vi "CameraSerialController_2024-04-21.vi"() -> (4 "图像时间戳":u32=16532020 format="%_32g")   [LabVIEW 2015]
uses:
  <vilib>/Instr/_visa.llb/VISA Configure Serial Port (Instr).vi
  MVCAMSDK.dll
  <vilib>/Analysis/NI_AALBase.lvlib
panel:
  out "实时循环时间":u32=16532020 format="%_32g"
  in  "平移前进 2":T1=TRUE
  in  "平移计数 2":u16
  in  "平移一次脉冲数 2":u16=20
  out "连接的字符串 2":string
  out "平移信号曲线 2":cluster{"Locations":dbl[], "Amplitudes":dbl[]}[](graph)
  out "光强图 4":dbl[](graph)
  out "variance 4":dbl caption="方差" format="%0.2f"
  out "光强图 3":dbl[](graph)
  out "variance 3":dbl caption="方差" format="%0.2f"
  out "连接的字符串":string
  out "转动信号曲线":cluster{"Locations":dbl[], "Amplitudes":dbl[]}[](graph)
  in  "平移回退":T1=TRUE
  in  "转动回退":T1=TRUE
  in  "转动计数":u16
  in  "转动一次脉冲数":u16=20
  in  "转动前进":T1=TRUE
  in  "平移一次脉冲数":u16=20
  in  "平移计数":u16
  out "variance 2":dbl caption="方差" format="%0.2f"
  in  "flow control (0:none)":u16(ring) caption="流控制（0:无）" items=["无", "XON/XOFF", "RTS/CTS", "XON/XOFF & RTS/CTS", "DTR/DSR", "XON/XOFF & DTR/DSR"]
  in  "stop bits (10: 1 bit)":u16=10 caption="停止位（10: 1位）"
  in  "奇偶 (0:none)":enum16{"None", "Odd", "Even", "Mark", "Space"}(ring) caption="奇偶（0:无）"
  in  "数据比特(默认8)":u16(ring)=8 items=["5"=5, "6"=6, "7"=7, "8"=8]
  in  "波特率(默认9600)":u32=9600
  in  "端口":refnum<visa-resource-name>="COM1"
  in  "平移前进":T1=TRUE
  out "泰伯距离数值":dbl[](array[numeric])=[15.393849374426454, 15.239052716055017, 15.197063981826837, 15.002070246239633]
  out "Locations":dbl[](array[numeric])=[10.438621227921368, 25.832470602347822, 41.07152331840284, 56.268587300229676, 71.27065754646931] caption="上面图像曲线波峰位置"
  out "平移信号曲线":cluster{"Locations":dbl[], "Amplitudes":dbl[]}[](graph)
  out "光强图 2":dbl[](graph)
  out "variance":dbl caption="方差" format="%0.2f"
  out "相机图像":T2(plugin-control)
  out "光强图":dbl[](graph)
  out "帧速":u32
  out "帧间耗时\n单位：（0.1ms）":u32
  in  "相机枚举":T3(ring)
  in  "自动曝光模式":bool=TRUE caption="软触发"
  in  "手动曝光模式":bool caption="软触发"
  in  "曝光时间，单位微秒":dbl=11000.0 format="%#_6f"
  in  "硬触发模式":bool caption="软触发"
  in  "软触发模式":bool caption="软触发"
  in  "连续模式":bool caption="软触发"
  in  "软触发一帧":bool caption="软触发"
  in  "读取自定义数据":bool
  out "从相机中读出的字符串(32字节)":string
  in  "写入自定义数据":bool
  in  "要写入相机的字符串(32字节)":string
  in  "拍照":bool
  in  "相机参数":bool=TRUE
  in  "Stop":bool
  in  "激活预览":bool=TRUE
  out "Image":T2(plugin-control)
  # "相机原生分辨率设置"
  # "写入自定义数据"
  # "触发设置"
  # "曝光设置"
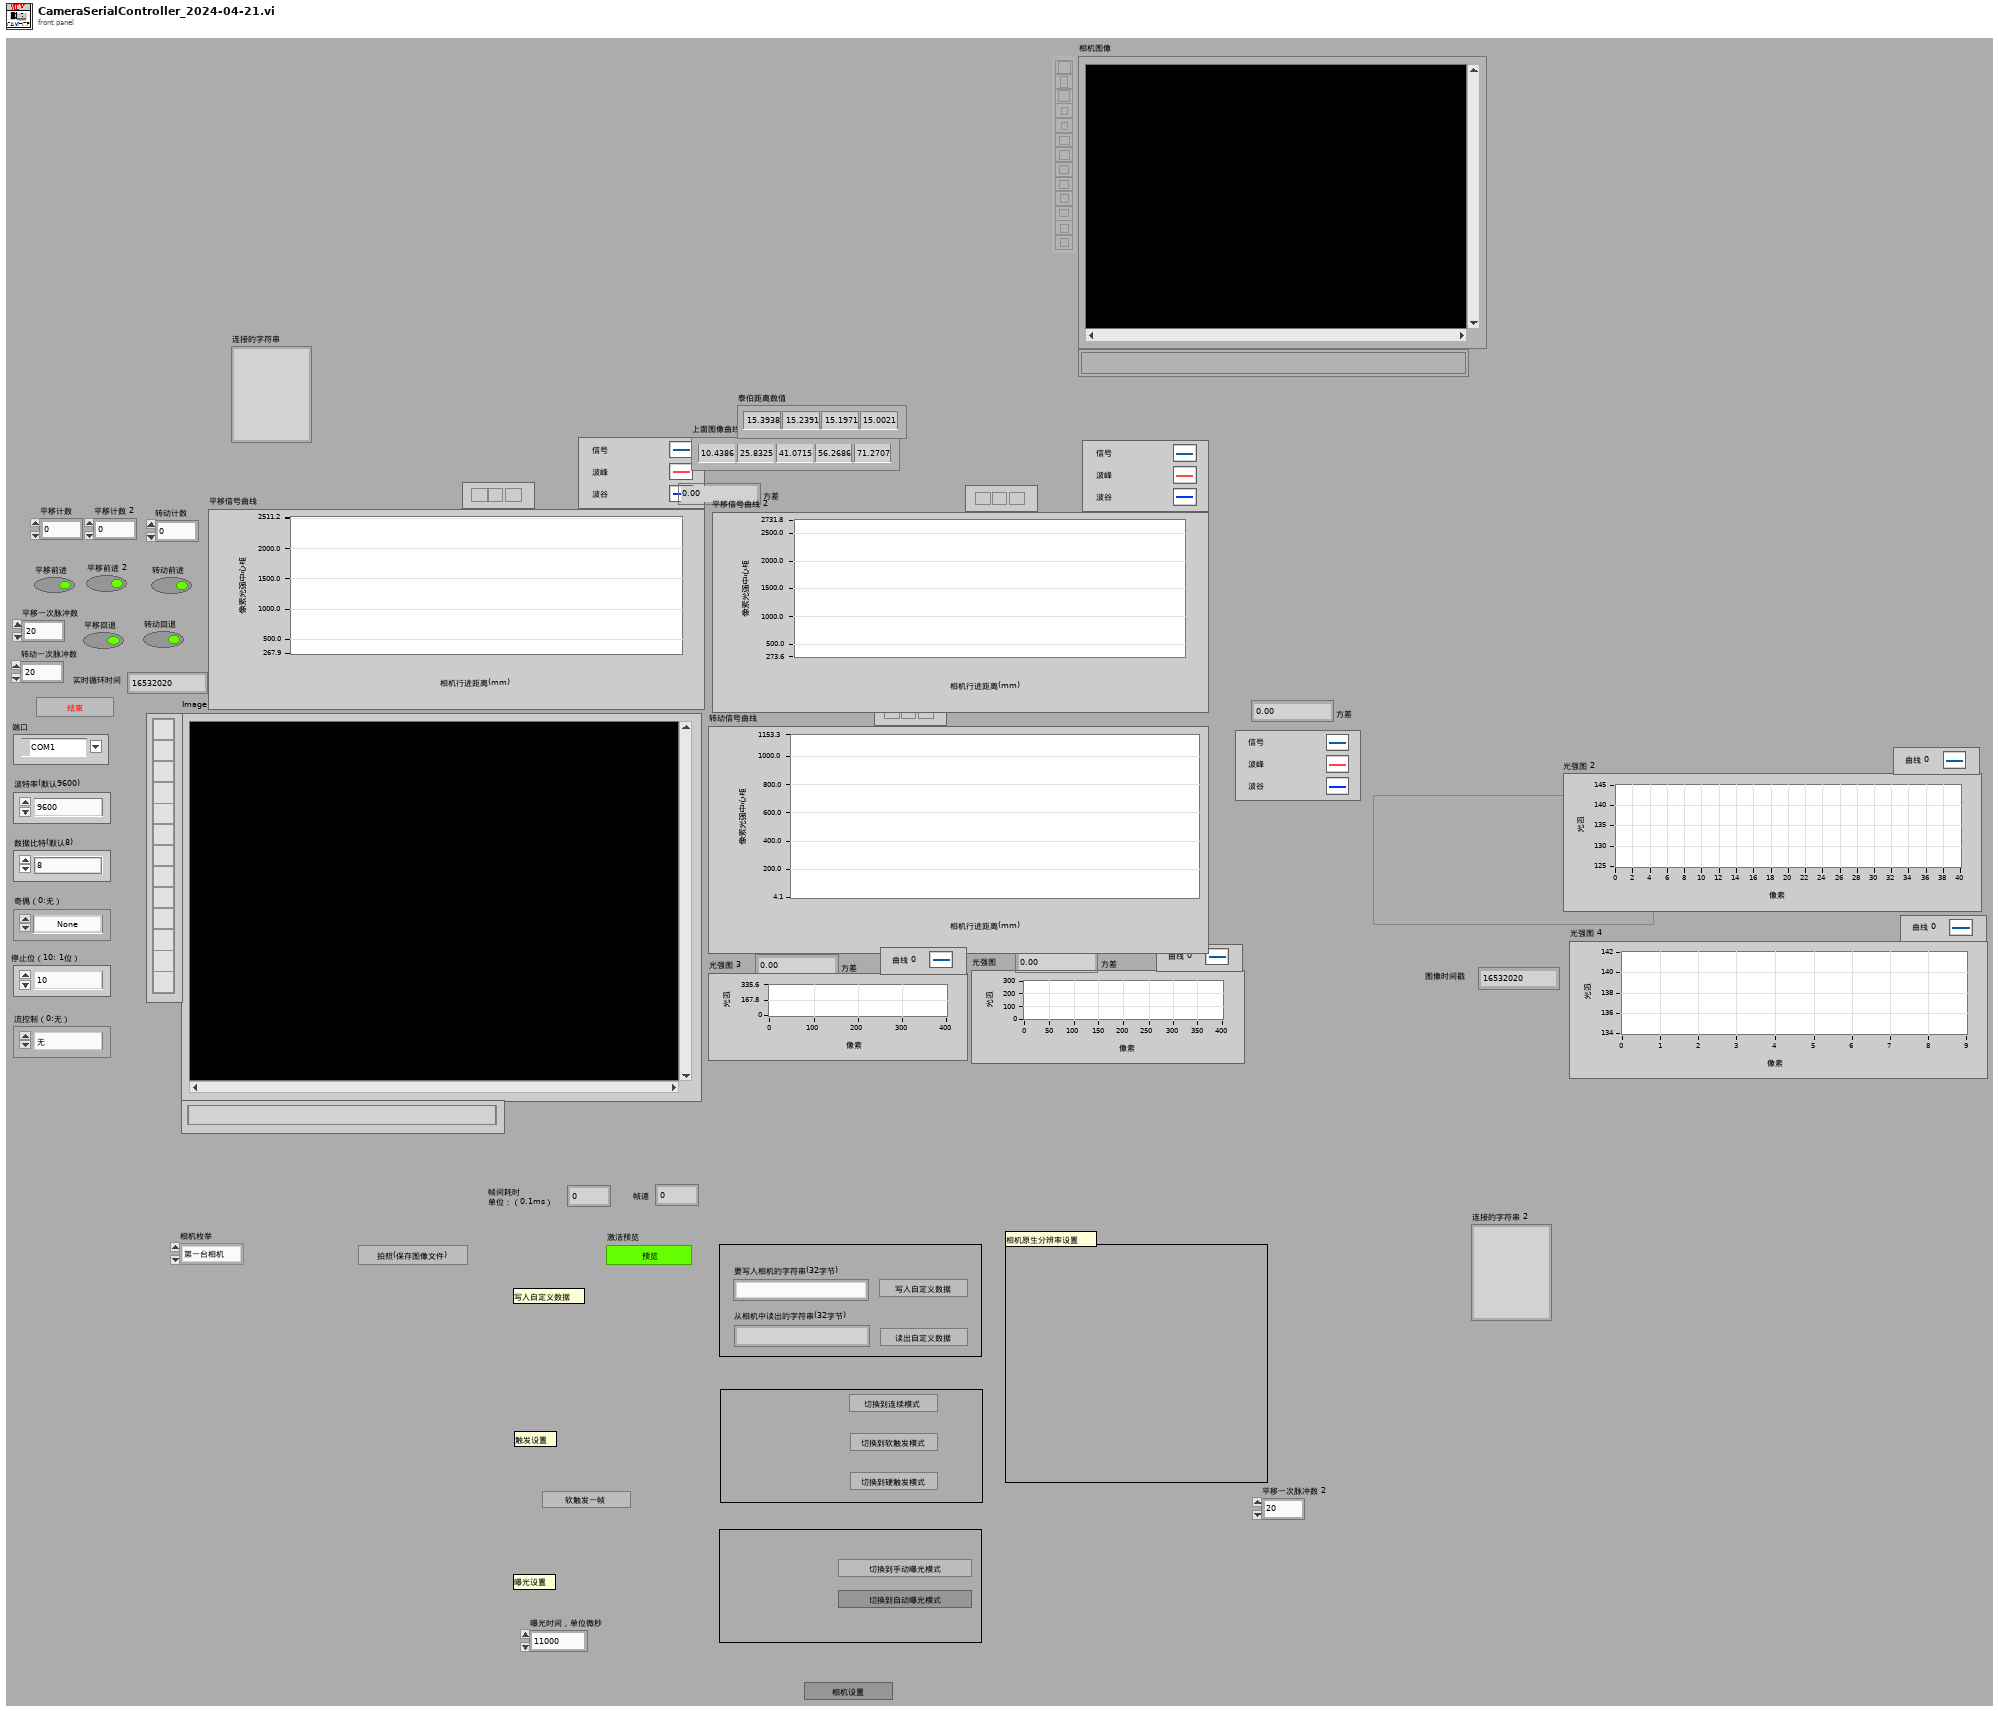
[diagram p1: front panel]
types:
  T1 = typedef "控件 1.ctl" = bool
  T2 = typedef "IMAQ Image.ctl" = refnum<image>
  T3 = enum16{"第一台相机", "第二台相机", "第三台相机", "第四台相机", "第五台相机"}
  T4 = typedef "Image Type" = u32
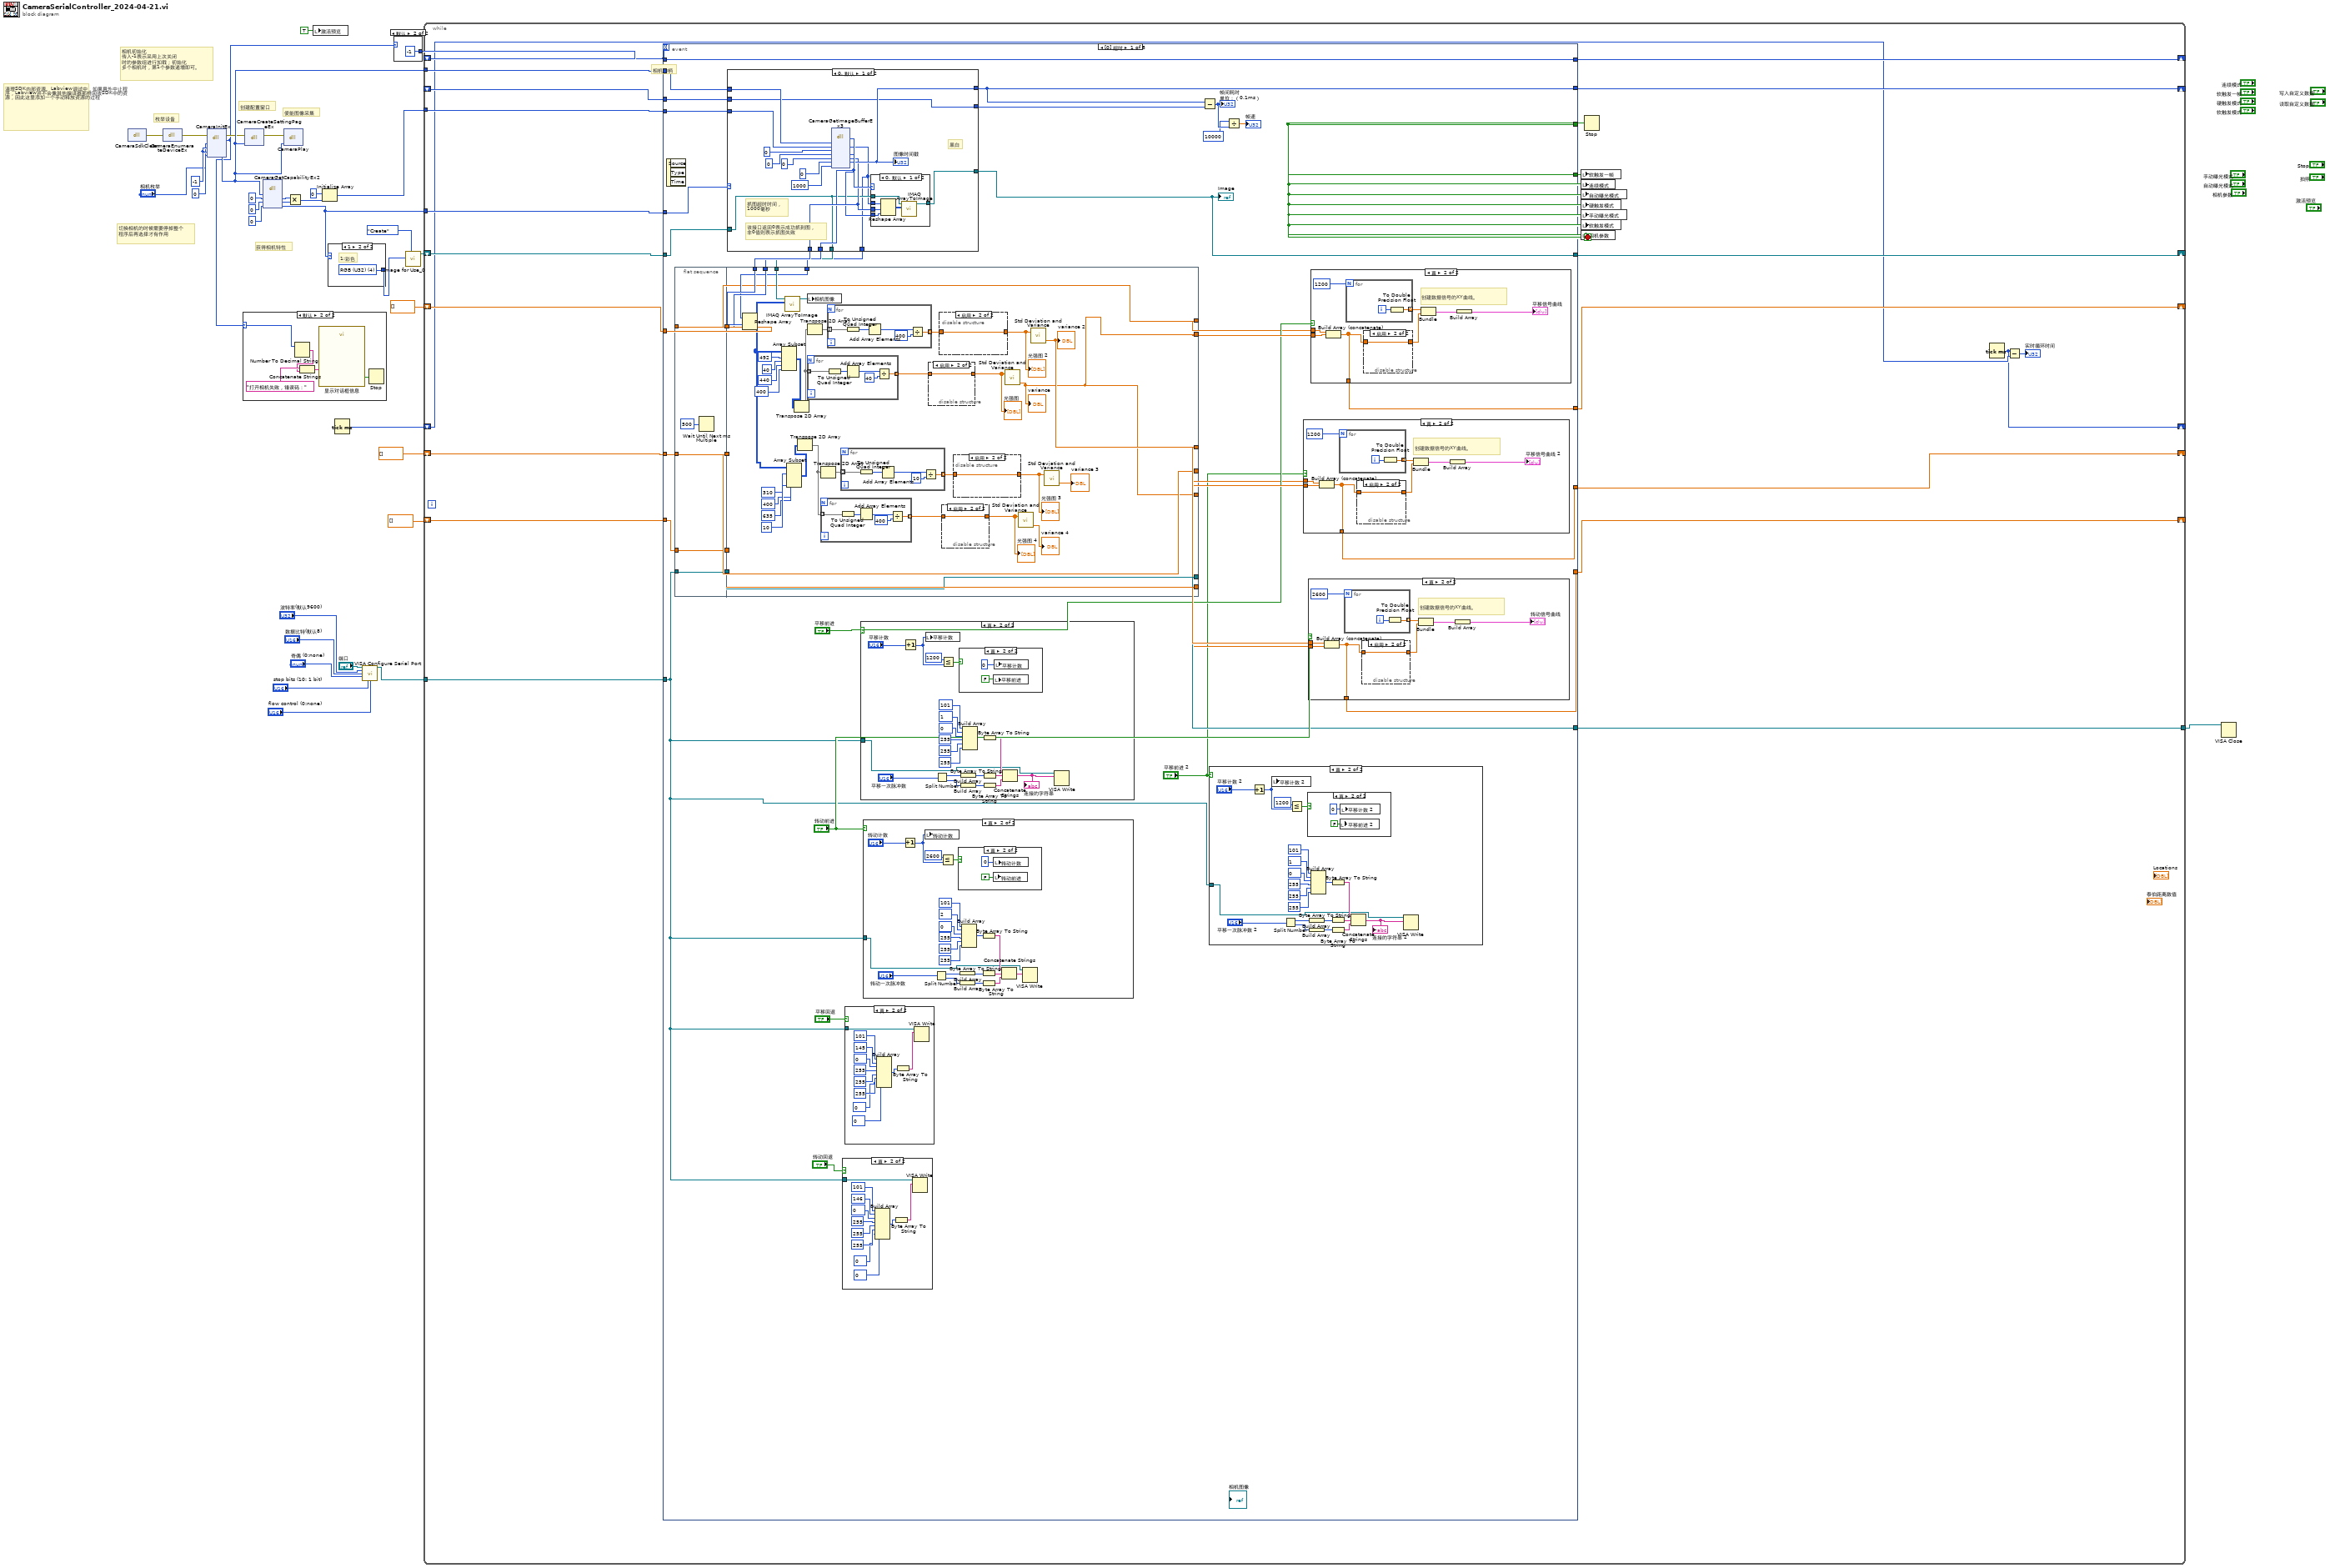
[diagram p0: block diagram]
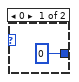
[diagram p2: hidden frame]
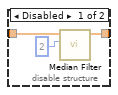
[diagram p7: hidden frame]
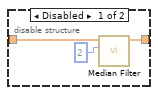
[diagram p8: hidden frame]
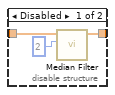
[diagram p9: hidden frame]
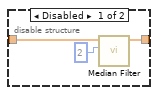
[diagram p10: hidden frame]
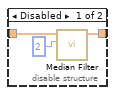
[diagram p11: hidden frame]
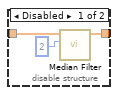
[diagram p13: hidden frame]
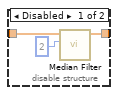
[diagram p15: hidden frame]
diagram:
  w32 = -1
  # "切换相机的时候需要停掉整个\n程序后再选择才有作用"
  # "清理SDK内部资源。Labview调试中，如果意外中止程序，Labview并不会像其他编译器那样回收SDK中的资源，因此这里添加一个手动释放资源的过程"
  # "使能图像采集"
  # "获得相机特性"
  # "创建配置窗口"
  # "相机初始化\n传入-1表示采用上次关闭\n时的参数组进行加载；初始化\n多个相机时，第1个参数递增即可。"
  # "枚举设备"
  n1 = dll-call lib="MVCAMSDK.dll" fn="CameraSdkClean"() -> (error out=w33:errorcluster)  [unwired: 4 in, 1 out]
  n2 = dll-call lib="MVCAMSDK.dll" fn="CameraEnumerateDeviceEx"(error in=w33) -> (error out=w30:errorcluster)  [unwired: 3 in, 1 out]
  n3 = dll-call lib="MVCAMSDK.dll" fn="CameraInitEx"(error in=w30, "相机索引值"="相机枚举", "参数加载方式"=w32, "要加载的参数组索引"=w32, "相机句柄"=0) -> (error out=w19:errorcluster, "返回类型"=w14:i32, "相机句柄"=w21:i32)  [unwired: 5 in, 1 out]
  n4 = case shown="默认" w14 {
    selector: w14 -> [_ w39]
    frame 0 {
    }
    frame Default {
      n5 = Number To Decimal String(number=w39) -> (decimal integer string=w36:string)  [unwired: 1 in]
      n6 = Concatenate Strings("打开相机失败，错误码：" ("字符串"), w36) -> (w38:string)
      n7 = call "显示对话框信息"("Message"=w38) -> ("结束"=w40:bool)  [unwired: 9 in, 1 out]
      n8 = Stop(stop? (T)=w40) -> ()
    }
  }
  n9 = dll-call lib="MVCAMSDK.dll" fn="CameraCreateSettingPageEx"(error in=w19, "相机句柄"=w21) -> (error out=w22:errorcluster)  [unwired: 4 in, 1 out]
  n10 = dll-call lib="MVCAMSDK.dll" fn="CameraGetCapabilityEx2"("相机句柄"=w21, "图像最大宽度"=0, "图像最大高度"=0, "是否是彩色相机(返回0:黑白;1:彩色)"=0) -> ("图像最大宽度"=w24:i32, "图像最大高度"=w23:i32, "是否是彩色相机(返回0:黑白;1:彩色)"=w18:i32)  [unwired: 5 in, 2 out]
  n11 = dll-call lib="MVCAMSDK.dll" fn="CameraPlay"(error in=w22, "相机句柄"=w21) -> ()  [unwired: 4 in, 2 out]
  n12 = Multiply(x=w24, y=w23) -> (x*y=w28:i32)
  n13 = local write "激活预览"(TRUE ("激活预览")) -> ()
  n14 = Initialize Array(0, w28) -> (w20:i32[])
  n15 = case shown="1" w18 {
    tunnel: [_ w41] -> w34
    frame 0, Default {
      # "0:黑白;"
    }
    frame 1 {
      w41 = T4 4 items=["Grayscale (U8)", "Grayscale (I16)", "Grayscale (SGL)", "Complex (CSG)", "RGB (U32)", "HSL (U32)", "RGB (U64)", "Grayscale (U16)"] ("Image Type")
      # "1:彩色"
    }
  }
  n16 = Tick Count (ms)() -> (millisecond timer value=w1:u32)
  n17 = call-poly "VISA Configure Serial Port"("VISA resource name"="端口", "baud rate (9600)"="波特率(默认9600)", "data bits (8)"="数据比特(默认8)", "parity (0:none)"="奇偶 (0:none)", "stop bits (10: 1 bit)"="stop bits (10: 1 bit)", "flow control (0:none)"="flow control (0:none)") -> ("VISA resource name out"=w6:refnum<visa-resource-name>)  [unwired: 8 in, 1 out]
  n18 = case shown="默认" w14 {
    tunnel: [0 -1] -> w13
    frame 0 {
    }
    frame Default {
    }
  }
  n19 = call "Image for Use_0.vi"("Command"=enum16{"Create", "Use", "Copy in", "Dispose"}."Create", "Image Type"=w34) -> ("Image out"=w17:T2)  [unwired: 8 in, 1 out]
  n20 = while {
    tunnel: w21 -> [w62]
    tunnel: w20 -> [w64]
    tunnel: w18 -> [w65]
    shift-right: [w61] -> _
    shift-left: w13 -> [w60]
    shift-right: [w58] -> _
    shift-left: w17 -> [w63]
    shift-right: [w57] -> _
    shift-left: _ -> [w56]
    tunnel: w6 -> [w54]
    tunnel: [w53] -> w5
    shift-right: [w51] -> _
    shift-left: dbl[] [] -> [w52]
    shift-right: [w50] -> _
    shift-left: dbl[] [] -> [w49]
    shift-right: [w47] -> _
    shift-left: dbl[] [] -> [w48]
    shift-right: [w44] -> _
    shift-left: w1 -> [w45]
    stop <- w55 stop-if-true
    # "相机句柄"
    n21 = event shown="[0] 超时" {
      selector: _ -> [_ _ _ _ _ _ _ _]
      dyn-events: _ -> [_ _ _ _ _ _ _ _]
      timeout: w60 -> [_ _ _ _ _ _ _ _]
      tunnel: [_ _ _ _ _ _ _ TRUE] -> w55
      tunnel: w64 -> [w103 _ _ _ _ _ _ _]
      tunnel: w65 -> [w102 _ _ _ _ _ _ _]
      tunnel: w62 -> [w104 _ w371 w389 w404 _ w418 w438]
      tunnel: w63 -> [w101 w364 w370 w388 w403 w408 w417 w436]
      tunnel: [w100 w365 w372 w390 w405 w409 w419 w439] -> w61
      tunnel: w60 -> [w100 _ w372 w390 w405 w409 w419 w439]
      tunnel: [_ _ _ _ _ _ _ FALSE] -> w59
      tunnel: [w99 w364 w370 w388 w403 w408 w417 w436] -> w58
      tunnel: [w96 w363 w369 w387 w402 w407 w416 w435] -> w57
      tunnel: w56 -> [w98 w363 w369 w387 w402 w407 w416 w435]
      tunnel: w54 -> [w66 _ _ _ _ _ _ _]
      tunnel: [w77 _ _ _ _ _ _ _] -> w53
      tunnel: w52 -> [w83 _ _ _ _ _ _ _]
      tunnel: [w86 _ _ _ _ _ _ _] -> w51
      tunnel: [w85 _ _ _ _ _ _ _] -> w50
      tunnel: w49 -> [w79 _ _ _ _ _ _ _]
      tunnel: [w74 _ _ _ _ _ _ _] -> w47
      tunnel: w48 -> [w71 _ _ _ _ _ _ _]
      event Timeout {
        n22 = event-data() -> ()  [unwired: 1 in, 3 out]
        n23 = flat-sequence {
          tunnel: w83 -> [w147]
          tunnel: [w147] -> w82
          tunnel: [w145] -> w80
          tunnel: w79 -> [w145]
          tunnel: [w144] -> w78
          tunnel: w66 -> [w144]
          tunnel: w71 -> [w143]
          tunnel: [w143] -> w70
          tunnel: w92 -> [w182]
          tunnel: w91 -> [w181]
          tunnel: w90 -> [w180]
          tunnel: w89 -> [w179]
          tunnel: [w149] -> w75
          tunnel: [w169] -> w68
          tunnel: w82 -> [w169]
          tunnel: [w168] -> w81
          tunnel: w80 -> [w168]
          tunnel: [w167] -> w77
          tunnel: w78 -> [w167]
          tunnel: [w151] -> w76
          tunnel: [w149] -> w73
          tunnel: w70 -> [w150]
          tunnel: [w150] -> w69
          frame #0 {
            n24 = Wait Until Next ms Multiple(millisecond multiple=u32 500 ("毫秒倍数")) -> ()  [unwired: 1 out]
          }
          frame #1 {
            n25 = Reshape Array(w179, w182, w181) -> (w156:u8[][])
            n26 = Array Subset(array=w156, index (row)=492 ("索引"), length (row)=40 ("长度"), index (col)=440 ("长度"), length (col)=400 ("索引")) -> (w153:u8[][])
            n27 = call "IMAQ ArrayToImage"("Image Pixels (U8)"=w156, "Image"=w180) -> ("Image Out"=w183:T2)  [unwired: 8 in, 1 out]
            n28 = Array Subset(array=w156, index (row)=310 ("索引"), length (row)=400 ("长度"), index (col)=635 ("长度"), length (col)=10 ("索引")) -> (w155:u8[][])
            n29 = Transpose 2D Array(2D array=w153) -> (transposed array=w152:u8[][])
            n30 = Transpose 2D Array(2D array=w155) -> (transposed array=w154:u8[][])
            n31 = local write "相机图像"(w183) -> ()
            n32 = Transpose 2D Array(2D array=w152) -> (transposed array=w176:u8[][])
            n33 = for {
              tunnel: w152 -> [w214] mode=indexing
              tunnel: [w212] -> w178 mode=indexing
              n34 = To Unsigned Quad Integer(1:w214) -> (0:w213:u64[])
              n35 = Add Array Elements(numeric array=w213) -> (sum=w215:u64)
              n36 = Divide(x=w215, y=u64 40) -> (x/y=w212:dbl)
            }
            n37 = Transpose 2D Array(2D array=w154) -> (transposed array=w160:u8[][])
            n38 = for {
              tunnel: w154 -> [w196] mode=indexing
              tunnel: [w194] -> w158 mode=indexing
              n39 = To Unsigned Quad Integer(1:w196) -> (0:w195:u64[])
              n40 = Add Array Elements(numeric array=w195) -> (sum=w197:u64)
              n41 = Divide(x=w197, y=u64 400) -> (x/y=w194:dbl)
            }
            n42 = for {
              tunnel: w176 -> [w205] mode=indexing
              tunnel: [w203] -> w177 mode=indexing
              n43 = To Unsigned Quad Integer(1:w205) -> (0:w204:u64[])
              n44 = Add Array Elements(numeric array=w204) -> (sum=w206:u64)
              n45 = Divide(x=w206, y=u64 400) -> (x/y=w203:dbl)
            }
            n46 = for {
              tunnel: w160 -> [w187] mode=indexing
              tunnel: [w185] -> w159 mode=indexing
              n47 = To Unsigned Quad Integer(1:w187) -> (0:w186:u64[])
              n48 = Add Array Elements(numeric array=w186) -> (sum=w188:u64)
              n49 = Divide(x=w188, y=u64 10) -> (x/y=w185:dbl)
            }
            n50 = disable-structure shown="启用" {
              disable-tunnel: w178 -> [w218 w219]
              disable-tunnel: [w216 w219] -> w175
              frame Disabled {
                n51 = call <vilib>:"Median Filter.vi"("left rank"=2, "X"=w218) -> ("Filtered X"=w216:dbl[])  [unwired: 8 in, 1 out]
              }
              frame Enabled {
              }
            }
            "光强图" <- w175
            n52 = disable-structure shown="启用" {
              disable-tunnel: w177 -> [w209 w210]
              disable-tunnel: [w207 w210] -> w174
              frame Disabled {
                n53 = call <vilib>:"Median Filter.vi"("left rank"=2, "X"=w209) -> ("Filtered X"=w207:dbl[])  [unwired: 8 in, 1 out]
              }
              frame Enabled {
              }
            }
            "光强图 2" <- w174
            n54 = disable-structure shown="启用" {
              disable-tunnel: w158 -> [w200 w201]
              disable-tunnel: [w198 w201] -> w161
              frame Disabled {
                n55 = call <vilib>:"Median Filter.vi"("left rank"=2, "X"=w200) -> ("Filtered X"=w198:dbl[])  [unwired: 8 in, 1 out]
              }
              frame Enabled {
              }
            }
            "光强图 4" <- w161
            n56 = disable-structure shown="启用" {
              disable-tunnel: w159 -> [w191 w192]
              disable-tunnel: [w189 w192] -> w162
              frame Disabled {
                n57 = call <vilib>:"Median Filter.vi"("left rank"=2, "X"=w191) -> ("Filtered X"=w189:dbl[])  [unwired: 8 in, 1 out]
              }
              frame Enabled {
              }
            }
            "光强图 3" <- w162
            n58 = call <vilib>:"Std Deviation and Variance.vi"("X"=w175) -> ("variance"=w149:dbl)  [unwired: 1 in, 2 out]
            "variance" <- w149
            n59 = call <vilib>:"Std Deviation and Variance.vi"("X"=w161) -> ("variance"=→"variance 4":dbl)  [unwired: 1 in, 2 out]
            n60 = call <vilib>:"Std Deviation and Variance.vi"("X"=w174) -> ("variance"=w151:dbl)  [unwired: 1 in, 2 out]
            "variance 2" <- w151
            n61 = call <vilib>:"Std Deviation and Variance.vi"("X"=w162) -> ("variance"=→"variance 3":dbl)  [unwired: 1 in, 2 out]
          }
        }
        n62 = case shown="0, 默认" w102 {
          tunnel: w103 -> [w332 w355]
          tunnel: w101 -> [w319 w354]
          tunnel: w104 -> [w324 w353]
          tunnel: [w325 w343] -> w99
          tunnel: [w323 w342] -> w96
          tunnel: w98 -> [w322 w341]
          tunnel: [w322 w341] -> w97
          tunnel: [w321 _] -> w92
          tunnel: [w320 _] -> w91
          tunnel: [w319 _] -> w90
          tunnel: [w318 _] -> w89
          frame 0, Default {
            # "黑白"
            # "该接口返回0表示成功抓到图，\n非0值则表示抓图失败"
            # "抓图超时时间，\n1000毫秒"
            n63 = dll-call lib="MVCAMSDK.dll" fn="CameraGetImageBufferEx3"("相机句柄"=w324, "图像数据缓冲区"=w332, "图像输出格式(0:8位灰度;1:24位彩色;2:32位彩色，3：BGR24彩色 4：BGRA32位彩色)"=0, "图像宽度"=0, "图像高度"=0, "时间戳(单位为100微秒)"=0, "抓图超时时间(毫秒)"=1000) -> ("返回类型"=w327:i32, "图像数据缓冲区"=w318:u8[], "图像宽度"=w320:i32, "图像高度"=w321:i32, "时间戳(单位为100微秒)"=w323:u32)  [unwired: 6 in, 2 out]
            "图像时间戳" <- w323
            n64 = case shown="0, 默认" w327 {
              tunnel: w318 -> [w338 _]
              tunnel: w319 -> [w335 w339]
              tunnel: w321 -> [w337 _]
              tunnel: w320 -> [w336 _]
              tunnel: [w333 w339] -> w325
              frame 0, Default {
                n65 = Reshape Array(w338, w337, w336) -> (w334:u8[][])
                n66 = call "IMAQ ArrayToImage"("Image Pixels (U8)"=w334, "Image"=w335) -> ("Image Out"=w333:T2)  [unwired: 8 in, 1 out]
              }
              frame -12 {
              }
            }
          }
          frame 1 {
            w345 = 0
            w346 = 0
            # "彩色"
            n67 = dll-call lib="MVCAMSDK.dll" fn="CameraGetImageBufferPriorityEx3"("相机句柄"=w353, "图像数据缓冲区"=w355, "图像输出格式(0:8位灰度;1:24位彩色;2:32位彩色)"=4, "图像宽度"=w345, "图像高度"=w346, "时间戳（单位为100微秒）"=0, "抓图超时时间(毫秒)"=1000, "取图优先级(0: 取最旧   1:取最新)"=1) -> ("返回类型"=w347:i32, "图像数据缓冲区"=w350:u32[], "图像宽度"=w348:i32, "图像高度"=w349:i32, "时间戳（单位为100微秒）"=w342:u32)  [unwired: 7 in, 2 out]
            n68 = case shown="0, 默认" w347 {
              tunnel: w350 -> [w360 _]
              tunnel: w354 -> [w359 w362]
              tunnel: w349 -> [w358 _]
              tunnel: w348 -> [w357 _]
              tunnel: w346 -> [_ _]
              tunnel: w345 -> [_ _]
              tunnel: [w356 w362] -> w343
              frame 0, Default {
                n69 = Reshape Array(w360, w358, w357) -> (w361:u32[][])
                n70 = call "IMAQ ArrayToColorImage"("Image Pixels (U32)"=w361, "Image"=w359) -> ("Image Out"=w356:T2)  [unwired: 3 in, 1 out]
              }
              frame -12 {
              }
            }
            n71 = local write "图像时间戳"(w342) -> ()
          }
        }
        "Image" <- w99
        n72 = case shown="真" "转动回退" {
          tunnel: w66 -> [_ w253]
          frame False {
          }
          frame True {
            n73 = Build Array(101, 146, 0, 255, 255, 255, 0, 0) -> (w254:i32[])
            n74 = Byte Array To String(unsigned byte array=w254) -> (string=w252:string)
            n75 = VISA Write(VISA resource name=w253, write buffer=w252) -> ()  [unwired: 1 in, 3 out]
          }
        }
        n76 = case shown="真" "平移回退" {
          tunnel: w66 -> [_ w264]
          frame False {
          }
          frame True {
            n77 = Build Array(101, 145, 0, 255, 255, 255, 0, 0) -> (w265:i32[])
            n78 = Byte Array To String(unsigned byte array=w265) -> (string=w263:string)
            n79 = VISA Write(VISA resource name=w264, write buffer=w263) -> ()  [unwired: 1 in, 3 out]
          }
        }
        n80 = case shown="真" "平移前进" {
          tunnel: w66 -> [_ w298]
          frame False {
          }
          frame True {
            n81 = Increment(x="平移计数") -> (x+1=w296:u16)
            n82 = local write "平移计数"(w296) -> ()
            n83 = Split Number(x="平移一次脉冲数") -> (hi(x)=w306:u8, lo(x)=w305:u8)
            n84 = Less Or Equal?(x=1200, y=w296) -> (x <= y?=w308:bool)
            n85 = case shown="真" w308 {
              frame False {
              }
              frame True {
                n86 = local write "平移前进"(T1 FALSE ("平移前进")) -> ()
                n87 = local write "平移计数"(u16 0 ("平移计数 2")) -> ()
              }
            }
            n88 = Build Array(w306) -> (w304:u8[])
            n89 = Build Array(w305) -> (w303:u8[])
            n90 = Build Array(101, 1, 0, 255, 255, 255) -> (w302:i32[])
            n91 = Byte Array To String(unsigned byte array=w302) -> (string=w301:string)
            n92 = Byte Array To String(unsigned byte array=w304) -> (string=w300:string)
            n93 = Byte Array To String(unsigned byte array=w303) -> (string=w299:string)
            n94 = Concatenate Strings(w301, w300, w299) -> (w295:string)
            "连接的字符串" <- w295
            n95 = VISA Write(VISA resource name=w298, write buffer=w295) -> ()  [unwired: 1 in, 3 out]
          }
        }
        n96 = case shown="真" "转动前进" {
          tunnel: w66 -> [_ w276]
          frame False {
          }
          frame True {
            n97 = Increment(x="转动计数") -> (x+1=w274:u16)
            n98 = local write "转动计数"(w274) -> ()
            n99 = Split Number(x="转动一次脉冲数") -> (hi(x)=w284:u8, lo(x)=w283:u8)
            n100 = Less Or Equal?(x=2600, y=w274) -> (x <= y?=w286:bool)
            n101 = case shown="真" w286 {
              frame False {
              }
              frame True {
                n102 = local write "转动前进"(T1 FALSE ("平移前进")) -> ()
                n103 = local write "转动计数"(u16 0 ("平移计数")) -> ()
              }
            }
            n104 = Build Array(w284) -> (w282:u8[])
            n105 = Build Array(w283) -> (w281:u8[])
            n106 = Build Array(101, 2, 0, 255, 255, 255) -> (w280:i32[])
            n107 = Byte Array To String(unsigned byte array=w280) -> (string=w279:string)
            n108 = Byte Array To String(unsigned byte array=w282) -> (string=w278:string)
            n109 = Byte Array To String(unsigned byte array=w281) -> (string=w277:string)
            n110 = Concatenate Strings(w279, w278, w277) -> (w273:string)
            n111 = VISA Write(VISA resource name=w276, write buffer=w273) -> ()  [unwired: 1 in, 3 out]
          }
        }
        n112 = Subtract(x=w96, y=w97) -> (x-y=w95:u32)
        "帧间耗时\n单位：（0.1ms）" <- w95
        n113 = case shown="真" "平移前进 2" {
          tunnel: w66 -> [_ w108]
          frame False {
          }
          frame True {
            n114 = Increment(x="平移计数 2") -> (x+1=w106:u16)
            n115 = local write "平移计数 2"(w106) -> ()
            n116 = Split Number(x="平移一次脉冲数 2") -> (hi(x)=w116:u8, lo(x)=w115:u8)
            n117 = Less Or Equal?(x=1200, y=w106) -> (x <= y?=w118:bool)
            n118 = case shown="真" w118 {
              frame False {
              }
              frame True {
                n119 = local write "平移前进 2"(T1 FALSE ("平移前进")) -> ()
                n120 = local write "平移计数 2"(u16 0 ("平移计数 2")) -> ()
              }
            }
            n121 = Build Array(w116) -> (w114:u8[])
            n122 = Build Array(w115) -> (w113:u8[])
            n123 = Build Array(101, 1, 0, 255, 255, 255) -> (w112:i32[])
            n124 = Byte Array To String(unsigned byte array=w112) -> (string=w111:string)
            n125 = Byte Array To String(unsigned byte array=w114) -> (string=w110:string)
            n126 = Byte Array To String(unsigned byte array=w113) -> (string=w109:string)
            n127 = Concatenate Strings(w111, w110, w109) -> (w105:string)
            "连接的字符串 2" <- w105
            n128 = VISA Write(VISA resource name=w108, write buffer=w105) -> ()  [unwired: 1 in, 3 out]
          }
        }
        n129 = Divide(x=u32 10000 ("帧间耗时"), y=w95) -> (x/y=→"帧速":dbl)
        n130 = case shown="真" "平移前进 2" {
          tunnel: w69 -> [w128 w131]
          tunnel: w73 -> [_ w129]
          tunnel: [w128 w130] -> w74
          frame False {
          }
          frame True {
            # "创建数据信号的XY曲线。"
            n131 = Build Array (concatenate)(w131, w129) -> (w130:dbl[])
            n132 = for {
              N: i64 1200 ("数值") -> [_]
              tunnel: [w137] -> w135 mode=indexing
              i -> [w138]
              n133 = To Double Precision Float(number=w138) -> (double precision float=w137:dbl)
            }
            n134 = disable-structure shown="启用" {
              disable-tunnel: w130 -> [w140 w142]
              disable-tunnel: [w139 w142] -> w134
              frame Disabled {
                n135 = call <vilib>:"Median Filter.vi"("left rank"=2, "X"=w140) -> ("Filtered X"=w139:dbl[])  [unwired: 8 in, 1 out]
              }
              frame Enabled {
              }
            }
            n136 = Bundle(w135, w134) -> (w132:cluster{dbl[], dbl[]})  [unwired: 1 in]
            n137 = Build Array(w132) -> (→"平移信号曲线 2":cluster{dbl[], dbl[]}[])
          }
        }
        n138 = case shown="真" "转动前进" {
          tunnel: w76 -> [_ w223]
          tunnel: w81 -> [w220 w222]
          tunnel: [w220 w221] -> w85
          frame False {
          }
          frame True {
            # "创建数据信号的XY曲线。"
            n139 = Build Array (concatenate)(w222, w223) -> (w221:dbl[])
            n140 = for {
              N: i64 2600 ("数值") -> [_]
              tunnel: [w229] -> w225 mode=indexing
              i -> [w230]
              n141 = To Double Precision Float(number=w230) -> (double precision float=w229:dbl)
            }
            n142 = disable-structure shown="启用" {
              disable-tunnel: w221 -> [w232 w234]
              disable-tunnel: [w231 w234] -> w226
              frame Disabled {
                n143 = call <vilib>:"Median Filter.vi"("left rank"=2, "X"=w232) -> ("Filtered X"=w231:dbl[])  [unwired: 8 in, 1 out]
              }
              frame Enabled {
              }
            }
            n144 = Bundle(w225, w226) -> (w228:cluster{dbl[], dbl[]})  [unwired: 1 in]
            n145 = Build Array(w228) -> (→"转动信号曲线":cluster{dbl[], dbl[]}[])
          }
        }
        n146 = case shown="真" "平移前进" {
          tunnel: w68 -> [w235 w237]
          tunnel: w75 -> [_ w238]
          tunnel: [w235 w236] -> w86
          frame False {
          }
          frame True {
            # "创建数据信号的XY曲线。"
            n147 = Build Array (concatenate)(w237, w238) -> (w236:dbl[])
            n148 = for {
              N: i64 1200 ("数值") -> [_]
              tunnel: [w244] -> w242 mode=indexing
              i -> [w245]
              n149 = To Double Precision Float(number=w245) -> (double precision float=w244:dbl)
            }
            n150 = disable-structure shown="启用" {
              disable-tunnel: w236 -> [w247 w249]
              disable-tunnel: [w246 w249] -> w241
              frame Disabled {
                n151 = call <vilib>:"Median Filter.vi"("left rank"=2, "X"=w247) -> ("Filtered X"=w246:dbl[])  [unwired: 8 in, 1 out]
              }
              frame Enabled {
              }
            }
            n152 = Bundle(w242, w241) -> (w239:cluster{dbl[], dbl[]})  [unwired: 1 in]
            n153 = Build Array(w239) -> (→"平移信号曲线":cluster{dbl[], dbl[]}[])
          }
        }
      }
      event "激活预览": Value Change {
        n154 = event-data() -> ("NewVal"=w366:bool)  [unwired: 1 in, 5 out]
        n155 = case shown="真" w366 {
          tunnel: [-1 0] -> w365
          frame False {
          }
          frame True {
          }
        }
      }
      event "连续模式", "软触发一帧", "硬触发模式", "软触发模式": Value Change {
        n156 = event-data() -> ("CtlRef"=w374:refnum<vi>)  [unwired: 1 in, 5 out]
        n157 = control-ref of="连续模式"() -> (w376:refnum<vi>)
        n158 = control-ref of="硬触发模式"() -> (w377:refnum<vi>)
        n159 = control-ref of="软触发模式"() -> (w378:refnum<vi>)
        n160 = control-ref of="软触发一帧"() -> (w379:refnum<vi>)
        n161 = Build Array ("创建数组")(w376, w377, w378, w379) -> (w375:refnum<vi>[])
        n162 = Search 1D Array(1D array=w375, element=w374) -> (index of element=w373:i32)  [unwired: 1 in]
        n163 = case shown="1" w373 {
          tunnel: w371 -> [w380 w382 w384 w386]
          frame 0, Default {
            # "连续模式"
            n164 = dll-call lib="MVCAMSDK.dll" fn="CameraSetTriggerMode"("相机句柄"=w380, "模式"=0) -> ()  [unwired: 6 in, 2 out]
          }
          frame 1 {
            # "硬触发模式"
            n165 = dll-call lib="MVCAMSDK.dll" fn="CameraSetTriggerMode"("相机句柄"=w382, "模式"=2) -> ()  [unwired: 6 in, 2 out]
          }
          frame 2 {
            # "软触发模式"
            n166 = dll-call lib="MVCAMSDK.dll" fn="CameraSetTriggerMode"("相机句柄"=w384, "模式"=1) -> ()  [unwired: 6 in, 2 out]
          }
          frame 3 {
            # "软触发一帧"
            n167 = dll-call lib="MVCAMSDK.dll" fn="CameraSoftTrigger"("相机句柄"=w386) -> ()  [unwired: 5 in, 2 out]
          }
        }
      }
      event "手动曝光模式", "自动曝光模式": Value Change {
        n168 = event-data() -> ("CtlRef"=w393:refnum<vi>)  [unwired: 1 in, 5 out]
        n169 = control-ref of="自动曝光模式"() -> (w391:refnum<vi>)
        n170 = control-ref of="手动曝光模式"() -> (w394:refnum<vi>)
        n171 = Build Array ("创建数组")(w394, w391) -> (w395:refnum<vi>[])
        n172 = Search 1D Array(1D array=w395, element=w393) -> (index of element=w392:i32)  [unwired: 1 in]
        n173 = case shown="0, 默认" w392 {
          tunnel: w389 -> [w396 w400]
          frame 0, Default {
            # "手动曝光模式"
            n174 = dll-call lib="MVCAMSDK.dll" fn="CameraSetAeState"("相机句柄"=w396, "曝光模式(0手动，1自动)"=0) -> (error out=w399:errorcluster)  [unwired: 6 in, 1 out]
            n175 = dll-call lib="MVCAMSDK.dll" fn="CameraSetExposureTime"(error in=w399, "相机句柄"=w396, "曝光时间，单位微秒"="曝光时间，单位微秒") -> ()  [unwired: 5 in, 2 out]
          }
          frame 1 {
            # "自动曝光模式"
            n176 = dll-call lib="MVCAMSDK.dll" fn="CameraSetAeState"("相机句柄"=w400, "曝光模式(0手动，1自动)"=1) -> ()  [unwired: 6 in, 2 out]
          }
        }
      }
      event "相机参数": Value Change {
        n177 = event-data() -> ()  [unwired: 1 in, 6 out]
        n178 = dll-call lib="MVCAMSDK.dll" fn="CameraShowSettingPage"("相机句柄"=w404, "状态"=TRUE) -> ()  [unwired: 6 in, 2 out]
      }
      event "拍照": Value Change {
        n179 = event-data() -> ()  [unwired: 1 in, 6 out]
        n180 = local read "Image"() -> (w410:T2)
        n181 = Format Date/Time String(time format string (%c)="%Y-%m-%d %H：%M：%S.bmp ") -> (date/time string=w414:string)  [unwired: 2 in]
        n182 = Concatenate Strings("c:\\", w414) -> (w411:string)
        n183 = String To Path(string=w411) -> (path=w413:path)
        n184 = call-poly "IMAQ Write File 2"("File Path"=w413, "Image"=w410) -> ()  [unwired: 8 in, 2 out]
      }
      event "写入自定义数据", "读取自定义数据": Value Change {
        n185 = event-data() -> ("CtlRef"=w421:refnum<vi>)  [unwired: 1 in, 5 out]
        n186 = control-ref of="读取自定义数据"() -> (w423:refnum<vi>)
        n187 = control-ref of="写入自定义数据"() -> (w422:refnum<vi>)
        n188 = Build Array ("创建数组")(w423, w422) -> (w424:refnum<vi>[])
        n189 = Search 1D Array(1D array=w424, element=w421) -> (index of element=w420:i32)  [unwired: 1 in]
        n190 = case shown="0, 默认" w420 {
          tunnel: w418 -> [w425 w432]
          frame 0, Default {
            n191 = Initialize Array(0, 32) -> (w429:i32[])
            n192 = dll-call lib="MVCAMSDK.dll" fn="CameraReadSN"("相机句柄"=w425, "序列号"=w429, "序列号级别，[0,1,2],0级为只读，1,2级可写"=1) -> ("序列号"=w427:u8[])  [unwired: 6 in, 2 out]
            n193 = Byte Array To String(unsigned byte array=w427) -> (string=→"从相机中读出的字符串(32字节)":string)
          }
          frame 1 {
            n194 = dll-call lib="MVCAMSDK.dll" fn="CameraWriteSN"("相机句柄"=w432, "序列号(固定为32个字节)"="要写入相机的字符串(32字节)", "序列号级别，[0,1,2]对应3级序列号，其中0级为只读，1,2级可写"=1) -> ()  [unwired: 7 in, 2 out]
          }
        }
      }
      event "Stop": Value Change {
        # "反初始化相机"
        n195 = event-data() -> ()  [unwired: 1 in, 6 out]
        n196 = dll-call lib="MVCAMSDK.dll" fn="CameraUnInit"("相机句柄"=w438) -> ()  [unwired: 5 in, 2 out]
      }
    }
    n197 = local write "软触发一帧"(w59) -> ()
    n198 = local write "连续模式"(w59) -> ()
    n199 = local write "自动曝光模式"(w59) -> ()
    n200 = local write "硬触发模式"(w59) -> ()
    n201 = local write "手动曝光模式"(w59) -> ()
    n202 = local write "软触发模式"(w59) -> ()
    n203 = local write "相机参数"(w59) -> ()
    n204 = Stop(stop? (T)=w55) -> ()
    n205 = Tick Count (ms)() -> (millisecond timer value=w44:u32)
    n206 = Subtract(x=w44, y=w45) -> (x-y=→"实时循环时间":u32)
  }
  n207 = VISA Close(VISA resource name=w5) -> ()  [unwired: 1 in, 1 out]
